vi "最小二乘法拟合圆.vi"(0 "x":dbl[](array[numeric]), 1 "y":dbl[](array[numeric])) -> (2 "拟合结果":T1, 3 "x":dbl, 4 "y":dbl)   [LabVIEW 2016]
uses:
  <vilib>/Analysis/baseanly.llb/Mean (DBL).vi
  <vilib>/Analysis/NI_AALBase.lvlib
  <vilib>/ptbypt/NI_PtbyPt.lvlib
panel:
  in  "簇":T1
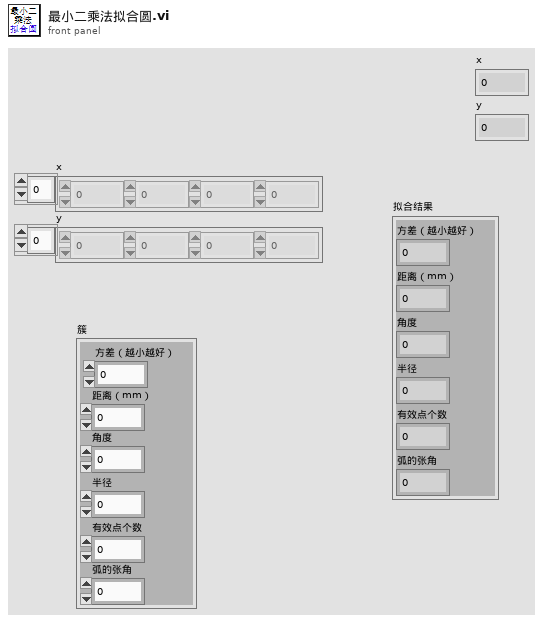
[diagram p1: front panel]
types:
  T1 = cluster{"方差（越小越好）":dbl, "距离（mm）":dbl, "角度":dbl, "半径":dbl, "有效点个数":i32, "弧的张角":dbl}
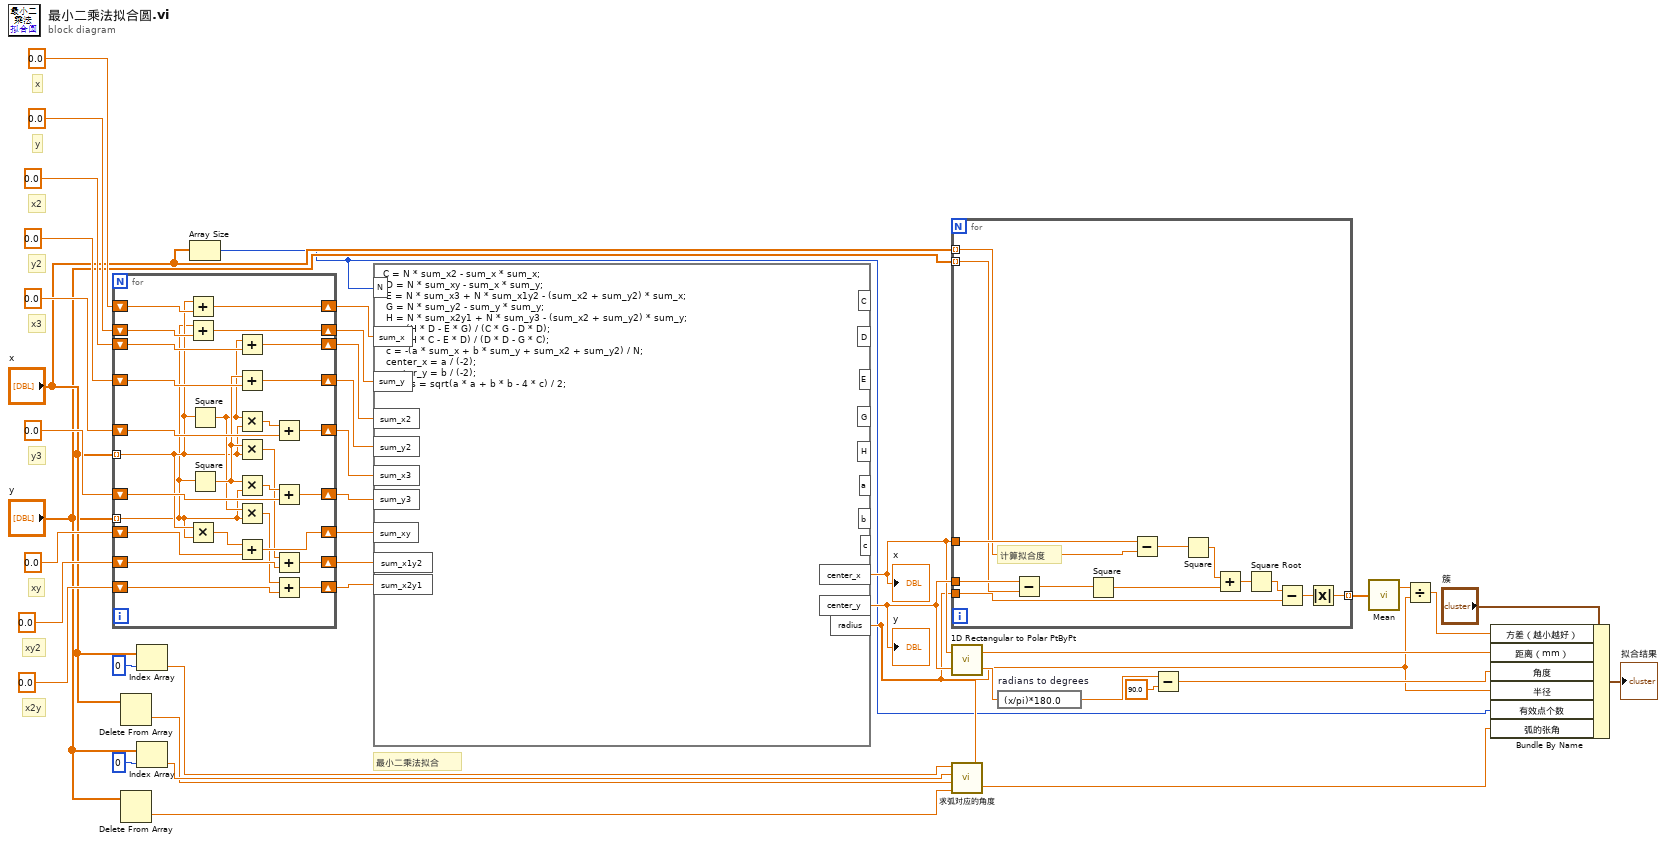
[diagram p0: block diagram]
diagram:
  # "最小二乘法拟合"
  # "x2y"
  # "xy2"
  # "xy"
  # "y3"
  # "x3"
  # "y2"
  # "x2"
  # "y"
  # "x"
  n1 = for {
    shift-right: [w68] -> w32
    shift-left: 0.0 -> [w67]
    shift-right: [w65] -> w31
    shift-left: 0.0 -> [w66]
    shift-right: [w63] -> w30
    shift-left: 0.0 -> [w64]
    shift-right: [w61] -> w29
    shift-left: 0.0 -> [w62]
    shift-right: [w58] -> w28
    shift-left: 0.0 -> [w59]
    shift-right: [w55] -> w27
    shift-left: 0.0 -> [w56]
    shift-right: [w52] -> w26
    shift-left: 0.0 -> [w53]
    shift-right: [w48] -> w25
    shift-left: 0.0 -> [w49]
    shift-right: [w44] -> w24
    shift-left: 0.0 -> [w45]
    tunnel: "x" -> [w43] mode=indexing
    tunnel: "y" -> [w42] mode=indexing
    n2 = Add(x=w43, y=w67) -> (x+y=w68:dbl)
    n3 = Add(x=w42, y=w66) -> (x+y=w65:dbl)
    n4 = Multiply(x=w43, y=w42) -> (x*y=w54:dbl)
    n5 = Square(x=w43) -> (x^2=w47:dbl)
    n6 = Square(x=w42) -> (x^2=w51:dbl)
    n7 = Add(x=w47, y=w64) -> (x+y=w63:dbl)
    n8 = Add(x=w51, y=w62) -> (x+y=w61:dbl)
    n9 = Multiply(x=w47, y=w43) -> (x*y=w60:dbl)
    n10 = Multiply(x=w51, y=w43) -> (x*y=w50:dbl)
    n11 = Multiply(x=w51, y=w42) -> (x*y=w57:dbl)
    n12 = Multiply(x=w47, y=w42) -> (x*y=w46:dbl)
    n13 = Add(x=w54, y=w53) -> (x+y=w52:dbl)
    n14 = Add(x=w60, y=w59) -> (x+y=w58:dbl)
    n15 = Add(x=w57, y=w56) -> (x+y=w55:dbl)
    n16 = Add(x=w50, y=w49) -> (x+y=w48:dbl)
    n17 = Add(x=w46, y=w45) -> (x+y=w44:dbl)
  }
  n18 = Delete From Array(array="x") -> (deleted portion=w16:dbl)  [unwired: 2 in, 1 out]
  n19 = Delete From Array(array="y") -> (deleted portion=w14:dbl)  [unwired: 2 in, 1 out]
  n20 = Index Array(array="x", index=0 ("索引")) -> (element=w20:dbl)
  n21 = Index Array(array="y", index=0 ("索引")) -> (element=w18:dbl)
  n22 = Array Size(array="x") -> (size(s)=w3:i32)
  n23 = formula code="C = N * sum_x2 - sum_x * sum_x;\n\tD = N * sum_xy - sum_x * sum_y;\n\tE = N * sum_x3 + N * sum_x1y2 - (sum_x2 + sum_y2) * sum_x;\n\tG = N * sum_y2 - sum_y * sum_y;\n\tH = N * sum_x2y1 + N * sum_y3 - (sum_x2 + sum_y2) * sum_y;\n\ta = (H * D - E * G) / (C * G - D * D);\n\tb = (H * C - E * D) / (D * D - G * C);\n\tc = -(a * sum_x + b * sum_y + sum_x2 + sum_y2) / N;\n\tcenter_x = a / (-2);\n\tcenter_y = b / (-2);\n\tradius = sqrt(a * a + b * b - 4 * c) / 2;"("sum_x"=w32, "sum_y"=w31, "sum_x2"=w30, "sum_y2"=w29, "sum_x3"=w28, "sum_y3"=w27, "sum_xy"=w26, "sum_x1y2"=w25, "sum_x2y1"=w24, "N"=w3) -> ("center_x"=w12:dbl, "center_y"=w13:dbl, "radius"=w4:dbl)  [unwired: 8 out]
  "x" <- w12
  "y" <- w13
  n24 = for {
    tunnel: w12 -> [w81]
    tunnel: w13 -> [w79]
    tunnel: w4 -> [w73]
    tunnel: [w71] -> w23 mode=indexing
    tunnel: "x" -> [w70] mode=indexing
    tunnel: "y" -> [w69] mode=indexing
    # "计算拟合度"
    n25 = Subtract(x=w79, y=w69) -> (x-y=w78:dbl)
    n26 = Square(x=w78) -> (x^2=w76:dbl)
    n27 = Subtract(x=w81, y=w70) -> (x-y=w80:dbl)
    n28 = Square(x=w80) -> (x^2=w77:dbl)
    n29 = Add(x=w77, y=w76) -> (x+y=w75:dbl)
    n30 = Square Root(x=w75) -> (sqrt(x)=w74:dbl)
    n31 = Subtract(x=w74, y=w73) -> (x-y=w72:dbl)
    n32 = Absolute Value(x=w72) -> (abs(x)=w71:dbl)
  }
  n33 = call <vilib>:"1D Rectangular to Polar PtByPt.vi"("y"=w13, "x"=w12) -> ("phase"=w10:dbl, "magnitude"=w6:dbl)
  n34 = call "求弧对应的角度.vi"("r"=w4, "y2"=w14, "x2"=w16, "y1"=w18, "x1"=w20) -> ("角度"=w2:dbl)
  n35 = expression code="(x/pi)*180.0" "radians to degrees"(w10) -> (w9:dbl)
  n36 = Subtract(x=w9, y=90.0) -> (x-y=w5:dbl)
  n37 = call-poly <vilib>:"Mean.vi"("X"=w23) -> ("mean"=w22:dbl)  [unwired: 1 out]
  n38 = Divide(x=w22, y=w4) -> (x/y=w7:dbl)
  n39 = Bundle By Name(cluster="簇", "方差（越小越好）"=w7, "距离（mm）"=w6, "角度"=w5, "半径"=w4, "有效点个数"=w3, "弧的张角"=w2) -> (→"拟合结果":T1)
